vi "Cypress LED Controller.vi"(8 "error in (no error)":errorcluster, 11 "Fire Ready within X RPM":dbl) -> ()   [LabVIEW 2011]
uses:
  Shared/Shooter Control Mode.ctl
  Shooter Global.vi
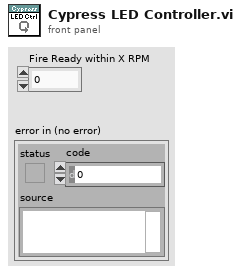
[diagram p1: front panel]
types:
  T1 = typedef "Shooter Control Mode.ctl" = enum16{"Key", "Mid Field", "Backfield", "Topspin", "Open Loop Control", "Off"}
  T2 = enum16{"Off", "Open Loop Control", "Closed Loop Control", "Top Spin"}
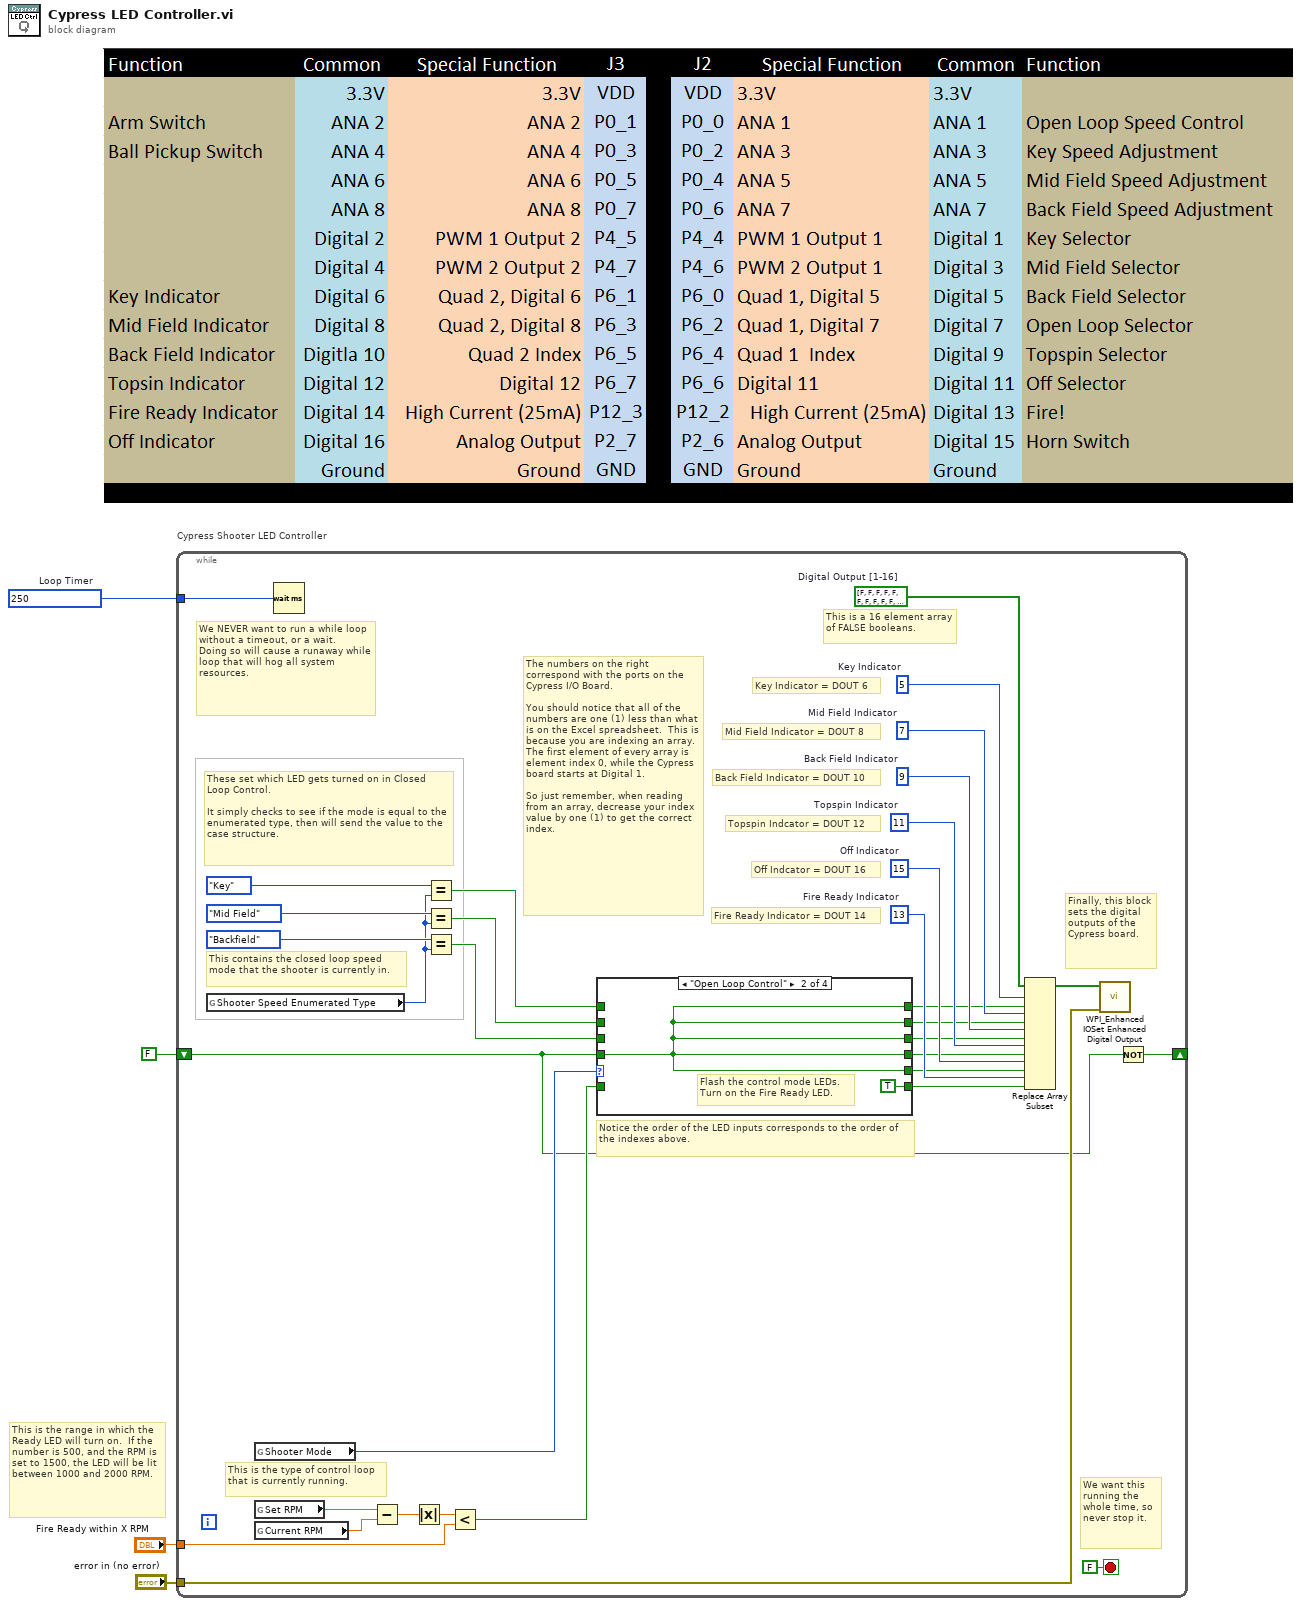
[diagram p0: block diagram]
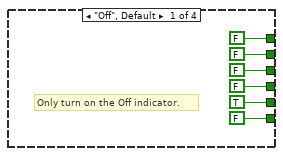
[diagram p2: hidden frame]
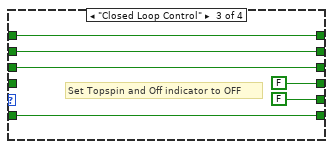
[diagram p3: hidden frame]
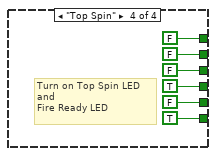
[diagram p4: hidden frame]
diagram:
  w2 = u32 250  # Loop Timer
  # "This is the range in which the Ready LED will turn on.  If the number is 500, and the RPM is set to 1500, the LED will be lit between 1000 and 2000 RPM."
  n1 = while "Cypress Shooter LED Controller" {
    tunnel: "Fire Ready within X RPM" -> [w24]
    tunnel: "error in (no error)" -> [w15]
    tunnel: w2 -> [w10]
    shift-right: [w6] -> _
    shift-left: FALSE -> [w5]
    stop <- FALSE stop-if-true
    w29 = 13  # Fire Ready Indicator
    w30 = 15  # Off Indicator
    w31 = 11  # Topspin Indicator
    w32 = 9  # Back Field Indicator
    w33 = 7  # Mid Field Indicator
    w34 = 5  # Key Indicator
    w36 = bool[] [FALSE, FALSE, FALSE, FALSE, FALSE, FALSE, FALSE, FALSE, FALSE, FALSE, FALSE, FALSE, FALSE, FALSE, FALSE, FALSE]  # Digital Output [1-16]
    # "We want this running the whole time, so never stop it."
    # "Finally, this block sets the digital outputs of the Cypress board."
    # "Notice the order of the LED inputs corresponds to the order of the indexes above."
    # "This contains the closed loop speed mode that the shooter is currently in."
    # "This is the type of control loop that is currently running."
    # "These set which LED gets turned on in Closed Loop Control.\n\nIt simply checks to see if the mode is equal to the enumerated type, then will send the value to the case structure."
    # "Fire Ready Indicator = DOUT 14"
    # "Off Indcator = DOUT 16"
    # "Topspin Indcator = DOUT 12"
    # "Back Field Indicator = DOUT 10"
    # "Mid Field Indicator = DOUT 8"
    # "Key Indicator = DOUT 6"
    # "The numbers on the right correspond with the ports on the Cypress I/O Board.\n\nYou should notice that all of the numbers are one (1) less than what is on the Excel spreadsheet.  This is because you are indexing an array.  The first element of every array is element index 0, while the Cypress board starts at Digital 1.\n\nSo just remember, when reading from an array, decrease your index value by one (1) to get the correct index."
    # "We NEVER want to run a while loop without a timeout, or a wait.  \nDoing so will cause a runaway while loop that will hog all system resources."
    # "This is a 16 element array of FALSE booleans."
    n2 = global read "Shooter Global.vi" "Shooter Speed Enumerated Type"() -> (w7:T1)
    n3 = global read "Shooter Global.vi" "Shooter Mode"() -> (w14:T2)
    n4 = global read "Shooter Global.vi" "Set RPM"() -> (w28:dbl)
    n5 = global read "Shooter Global.vi" "Current RPM"() -> (w27:dbl)
    n6 = Wait (ms)(milliseconds to wait=w10) -> ()  [unwired: 1 out]
    n7 = Subtract(x=w28, y=w27) -> (x-y=w26:dbl)
    n8 = Absolute Value(x=w26) -> (abs(x)=w25:dbl)
    n9 = Equal?(x=Shooter_Control_Mode."Key" ("y"), y=w7) -> (x = y?=w22:bool)
    n10 = Equal?(x=Shooter_Control_Mode."Mid Field" ("y"), y=w7) -> (x = y?=w20:bool)
    n11 = Equal?(x=Shooter_Control_Mode."Backfield" ("y"), y=w7) -> (x = y?=w18:bool)
    n12 = Less?(x=w25, y=w24) -> (x < y?=w11:bool)
    n13 = case shown="\"Open Loop Control\"" w14 {
      tunnel: [FALSE w45 w51 FALSE] -> w23
      tunnel: w22 -> [_ _ w51 _]
      tunnel: [FALSE w45 w50 FALSE] -> w21
      tunnel: w20 -> [_ _ w50 _]
      tunnel: [FALSE w45 w49 FALSE] -> w19
      tunnel: w18 -> [_ _ w49 _]
      tunnel: [FALSE w45 FALSE TRUE] -> w17
      tunnel: [TRUE w45 FALSE FALSE] -> w16
      tunnel: w5 -> [_ w45 _ _]
      tunnel: [FALSE TRUE w46 TRUE] -> w12
      tunnel: w11 -> [_ _ w46 _]
      frame "Off", Default {
        # "Only turn on the Off indicator."
      }
      frame "Open Loop Control" {
        # "Flash the control mode LEDs.\nTurn on the Fire Ready LED."
      }
      frame "Closed Loop Control" {
        # "Set Topspin and Off indicator to OFF"
      }
      frame "Top Spin" {
        # "Turn on Top Spin LED \nand \nFire Ready LED"
      }
    }
    n14 = Replace Array Subset(array=w36, new element #1=w23, index #1=w34, new element #2=w21, index #2=w33, new element #3=w19, index #3=w32, new element #4=w17, index #4=w31, new element #5=w16, index #5=w30, new element #6=w12, index #6=w29) -> (w35:bool[])
    n15 = call <vilib>:"WPI_Enhanced IOSet Enhanced Digital Output.vi"("error in (no error)"=w15, "Digital Output [1-16]"=w35) -> ()  [unwired: 9 in, 1 out]
    n16 = Not(x=w5) -> (.not. x?=w6:bool)
  }
